vi "changeState.vi"(8 "error in (no error)":errorcluster, 10 "detailedState":T1, 11 "Model in":refnum<class "Model.lvclass">) -> (0 "error out":errorcluster, 3 "Model out":refnum<class "Model.lvclass">)   [LabVIEW 2016, in "Model.lvclass"]
doc: "Changes the detailed state to the value of newState and publishes the new state."
uses:
  Model.lvclass
  ts_sallv_exa/DataTypes/logevent_DetailedState.ctl
  Typedefs/PubDataSignals.ctl
  Model.lvclass/Model.ctl
  Typedefs/EXATypedefs.lvlib
  ts_sallv_exa/SALLV_EXA.lvlib
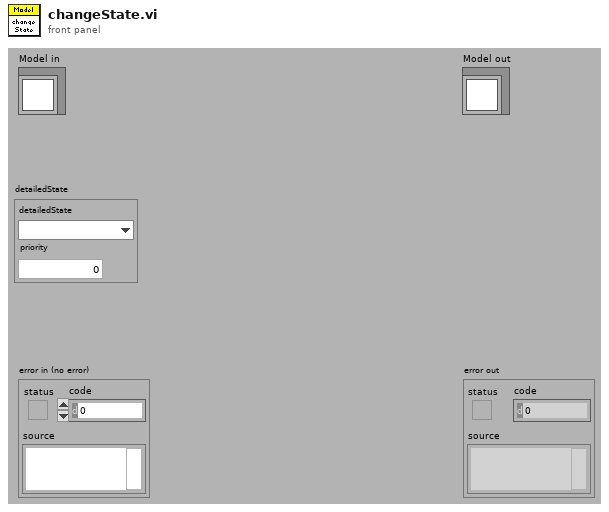
[diagram p1: front panel]
types:
  T1 = typedef "SALLV_EXA.lvlib/logevent_DetailedState.ctl" = cluster{"detailedState":enum16{"", " DisabledState", "EnabledState", "FaultState", "OfflineState", "StandbyState"}, "priority":i32}
  T2 = typedef "EXATypedefs.lvlib/PubDataSignals.ctl" = enum16{"DetailedState", "ErrorCode", "Heartbeat", "LoopTime_ms", "LoopTimeOutOfRange", "RejectedCommand", "SummaryState", "Timestamp", "SettingVersions", "AppliedSettingsMatchStart"}
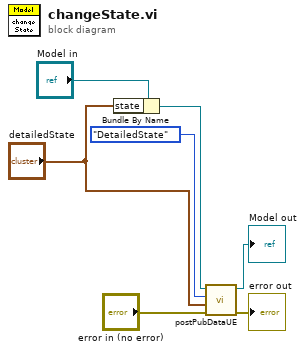
[diagram p0: block diagram]
diagram:
  n1 = Bundle By Name(cluster="Model in", "state"="detailedState") -> (w5:refnum<class "Model.lvclass">)
  n2 = call "postPubDataUE.vi"("error in (no error)"="error in (no error)", "value"="detailedState", "pubDataSV"=PubDataSignals."DetailedState", "Model in"=w5) -> ("error out"=→"error out":errorcluster, "Model out"=→"Model out":refnum<class "Model.lvclass">)  [unwired: 6 in]
